vi "RSZVB Get External Signal Source AUX.vi"(8 "error in (no error)":errorcluster {"code" format="%.0x"}, 9 "Channel (1)":i32=1, 11 "VISA session":refnum<visa-resource-name>) -> (0 "error out":errorcluster {"code" format="%.0x"}, 2 "External Signal Source":i32, 3 "dup VISA session":refnum<visa-resource-name>)   [LabVIEW 2011]
doc: "Queries an external generator as a signal source for the Aux LO signal in a vector mixer measurement (option R&S ZVA-K5). The Aux LO signal is fed to the MEAS and REF mixers.\n\nRemote-control command(s):\n[SENSe<Ch>:]FREQuency:CONVersion:MIXer:AEXTernal?"
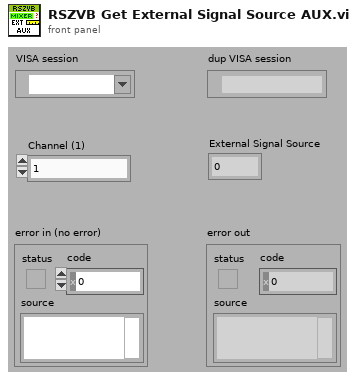
[diagram p1: front panel]
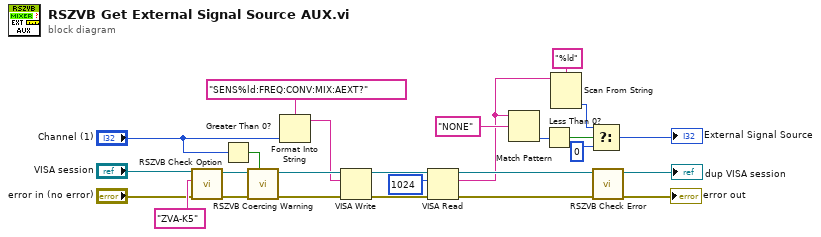
[diagram p0: block diagram]
diagram:
  n1 = call "RSZVB Check Option.vi"("error in (no error)"="error in (no error)", "Options"="ZVA-K5", "VISA session"="VISA session") -> ("error out"=w7:errorcluster, "dup VISA session"=w8:refnum<visa-resource-name>)  [unwired: 7 in]
  n2 = Greater Than 0?(x="Channel (1)") -> (x > 0?=w24:bool)
  n3 = call "RSZVB Coercing Warning.vi"("In Range?"=w24, "error in (no error)"=w7, "VISA session"=w8) -> ("error out"=w25:errorcluster, "dup VISA session"=w26:refnum<visa-resource-name>)  [unwired: 7 in]
  n4 = Format Into String(format string="SENS%ld:FREQ:CONV:MIX:AEXT?", "Channel (1)") -> (resulting string=w17:string)  [unwired: 2 in, 1 out]
  n5 = VISA Write(VISA resource name=w26, write buffer=w17, error in (no error)=w25) -> (VISA resource name out=w21:refnum<visa-resource-name>, error out=w22:errorcluster)  [unwired: 1 out]
  n6 = VISA Read(VISA resource name=w21, byte count=u32 1024 ("byte count (0)"), error in (no error)=w22) -> (VISA resource name out=w19:refnum<visa-resource-name>, read buffer=w11:string, error out=w20:errorcluster)  [unwired: 1 out]
  n7 = Match Pattern(string=w11, regular expression="NONE") -> (offset past match=w15:i32)  [unwired: 1 in, 3 out]
  n8 = Less Than 0?(x=w15) -> (x < 0?=w14:bool)
  n9 = Scan From String(format string="%ld", input string=w11) -> (output 1=w10:i32)  [unwired: 3 in, 3 out]
  n10 = Select(t=w10, s=w14, f=0 ("byte count (0)")) -> (s? t:f=→"External Signal Source":i32)
  n11 = call "RSZVB Check Error.vi"("error in (no error)"=w20, "VISA session"=w19) -> ("error out"=→"error out":errorcluster, "dup VISA session"=→"dup VISA session":refnum<visa-resource-name>)  [unwired: 8 in]
